vi "TryUpdateGyroSBIT.vi"   [LabVIEW 2018]
uses:
  <vilib>/Platform/TimedLoop/XDataNode/timing_clust.ctl
  <vilib>/Platform/TimedLoop/XDataNode/nitl_modes.ctl
  <vilib>/Platform/TimedLoop/XDataNode/wakeup.ctl
  Telemetry/TelemetryDataTypes.ctl
  Telemetry/TelemetryUpdateModes.ctl
  Telemetry/TelemetryFields.ctl
  <vilib>/rvi/Emulation/niFpgaEmulationIsFPGAContextNoSignature.vi
  <vilib>/rvi/Emulation/niFpgaSctlEmulationGetInTimedLoop.vi
  <vilib>/rvi/errors/niFpgaSetErrorForExecOnDevCompSimple.vi
  <vilib>/rvi/eio/common/nirviEmuReportErrorAndStop.vi
  <vilib>/rvi/DataTransferAndStorage/Container/Common/niFpgaContainerGetUniqueNameForEmu.vi
  <vilib>/rvi/FIFO/Fifo_Resource/nirvififoEmulationSetSize.vi
  <vilib>/rvi/FIFO/Fifo_Resource/nirviFifoEmulationQueueMgr.vi
  <instcachedir>/0/nirviFifoEmulationQueueMgr_E5CAEC123FF24DC58D834DCA3CDAA9B5.lvgen/nirviFifoEmulationQueueMgr_E5CAEC123FF24DC58D834DCA3CDAA9B5_009.vi
  <vilib>/Utility/error.llb/Clear Errors.vi
  <vilib>/rvi/FIFO/Fifo_Resource/nirvififoEmulationCreateLock.vi
  <vilib>/rvi/Emulation/niFpgaProcessEmulError.vi
  <vilib>/rvi/FIFO/Fifo_Resource/nirvififoEmulationObtainLock.vi
  <vilib>/rvi/FIFO/Fifo_Resource/nirvififoEmulationReleaseLock.vi
  <vilib>/rvi/occurrence/nirviWaitOnOccurrenceBase.vi
  <vilib>/rvi/errors/nirviReportUnexpectedCaseInternalError.vi
  <vilib>/rvi/errors/nirviReportUnexpectedCaseInternalError (U32).vi
  <vilib>/rvi/Emulation/niFpgaEmulationReportErrorSimple.vi
  <vilib>/rvi/Emulation/niFpgaGetClockAttributes.vi
  <vilib>/rvi/Emulation/niFpgaCriticalErrorInLSC.vi
  <instcachedir>/0/nirviFifoEmulationQueueMgr_E5CAEC123FF24DC58D834DCA3CDAA9B5.lvgen/nirviFifoEmulationQueueMgr_E5CAEC123FF24DC58D834DCA3CDAA9B5_007.vi
  <vilib>/rvi/FIFO/Fifo_Resource/nirvififoEmulationDetermineInputValidOut.vi
  <vilib>/rvi/Memory/Memory_Emulation/niFpgaMemoryEmulationCacheClearOnFirstRun.vi
  <vilib>/rvi/Memory/Memory_Emulation/nirvimemoryEmulationManagerCache_MakeExclusive.vi
  <vilib>/rvi/Memory/Memory_Emulation/niFpgaMemoryEmulationValidateCache.vi
  <vilib>/rvi/Memory/Memory_Emulation/nirvimemoryEmulationManagerCache_InsertValue.vi
  <vilib>/rvi/Memory/Memory_Emulation/nirvimemoryEmulationManagerCache_ReleaseExclusive.vi
  <vilib>/rvi/Memory/Memory_Emulation/nirvimemoryEmulationManagerCache_GetValue.vi
  <vilib>/rvi/Memory/Memory_Emulation/nirvimemoryEmulationManagerCache_SetValue.vi
  <vilib>/rvi/DataTransferAndStorage/Container/XNode/niFpgaContainer.xnode
  <vilib>/rvi/FIFO/Fifo_Resource/nirvififoEmulationRead.vi
  <vilib>/Platform/TimedLoop/XDataNode/XDataNode.xnode
  <vilib>/rvi/FIFO/Fifo_Resource/nirvififoEmulationWrite.vi
  <vilib>/rvi/DataTransferAndStorage/Register/Emulation/niFpgaRegisterEmulation.vi
  <vilib>/Platform/TimedLoop/XDataNode/XDNodeRunTimeDep.lvlib
types:
  T1 = cluster{"Timestamp":u64, "TxBytes":u64, "RxBytes":u64, "TxFrames":u64, "RxFrames":u64, "BIT0":u8, "BIT1":u8, "BIT2":u8, "BIT3":u8, "BIT4":u8, "BIT5":u8}
  T2 = typedef "TelemetryFields.ctl" = enum16{"None", "InclinometerTxBytes", "InclinometerRxBytes", "InclinometerTxFrames", "InclinometerRxFrames", "InclinometerErrorTimestamp", "InclinometerErrorCode", "InclinometerSampleTimestamp", "InclinometerAngleRaw", "DisplacementTxBytes", "DisplacementRxBytes", "DisplacementTxFrames", "DisplacementRxFrames", "DisplacementErrorTimestamp", "DisplacementErrorCode", "DisplacementSampleTimestamp", "DisplacementRaw1", "DisplacementRaw2", "DisplacementRaw3", "DisplacementRaw4", "DisplacementRaw5", "DisplacementRaw6", "DisplacementRaw7", "DisplacementRaw8", "AccelerometerSampleCount", "AccelerometerSampleTimestamp", "AccelerometerRaw1", "AccelerometerRaw2", "AccelerometerRaw3", "AccelerometerRaw4", "AccelerometerRaw5", "AccelerometerRaw6", "AccelerometerRaw7", "AccelerometerRaw8", "GyroTxBytes", "GyroRxBytes", "GyroTxFrames", "GyroRxFrames", "GyroErrorTimestamp", "GyroErrorCode", "GyroSampleTimestamp", "GyroRawX", "GyroRawY", "GyroRawZ", "GyroStatus", "GyroSequenceNumber", "GyroTemperature", "GyroBITTimestamp", "GyroBIT0", "GyroBIT1", "GyroBIT2", "GyroBIT3", "GyroBIT4", "GyroBIT5", "GyroBIT6", "GyroBIT7", "DigitalInputSampleCount", "DigitalInputTimestamp", "DigitalInputStates", "DigitalOutputSampleCount", "DigitalOutputTimestamp", "DigitalOutputStates", "PowerSupplySampleCount", "PowerSupplyTimestamp", "PowerSupplyStates", "Modbus1ErrorFlags", "Modbus1TxByteCount", "Modbus1TxFrameCount", "Modbus1RxByteCount", "Modbus1RxFrameCount", "Modbus2ErrorFlags", "Modbus2TxByteCount", "Modbus2TxFrameCount", "Modbus2RxByteCount", "Modbus2RxFrameCount", "Modbus3ErrorFlags", "Modbus3TxByteCount", "Modbus3TxFrameCount", "Modbus3RxByteCount", "Modbus3RxFrameCount", "Modbus4ErrorFlags", "Modbus4TxByteCount", "Modbus4TxFrameCount", "Modbus4RxByteCount", "Modbus4RxFrameCount"}
  T3 = typedef "TelemetryUpdateModes.ctl" = enum8{"=", "+", "-", "|"}
  T4 = typedef "TelemetryDataTypes.ctl" = enum8{"U8", "U16", "U32", "U64", "I8", "I16", "I32", "I64", "SGL"}
  T5 = typedef "XDNodeRunTimeDep.lvlib/timing_clust.ctl" = cluster{"Expected End [f-1]":u64, "Actual End [f-1]":u64, "Finished Late? [f-1]":bool, "Expected End [i-1]":u64, "Actual End [i-1]":u64, "Finished Late? [i-1]":bool, "Expected Start [i]":u64, "Actual Start [i]":u64, "Expected Start [f]":u64, "Actual Start [f]":u64, "Source Name":string, "Structure Name":string, "Period":i64, "Deadline":i64, "Offset":i64, "Start":i64, "Priority":i32, "Timeout":i32, "Mode":T6, "Wakeup Reason":T7, "Error":errorcluster, "Source Type":string, "Secondary Source Type":string, "Global End Time":u64, "Global Start Time":u64, "Frame Duration":u64, "Iteration Duration":u64, "Assigned CPU":i32, "I/O Scan Engine Mode":u32}
  T6 = typedef "XDNodeRunTimeDep.lvlib/nitl_modes.ctl" = enum32{"No Change", "Process missed periods, maintain original phase", "Discard missed periods, maintain original phase", "Process missed periods, ignore original phase", "Discard missed periods, ignore original phase"}
  T7 = typedef "XDNodeRunTimeDep.lvlib/wakeup.ctl" = enum32{"Normal", "Aborted", "Asynchronous wakeup", "Timing source error", "Timed loop error", "Timeout"}
  T8 = typedef "TelemetryUpdateData.ctl" = cluster{"DataType":T4, "Mode":T3, "Field":T2, "Data":u64}
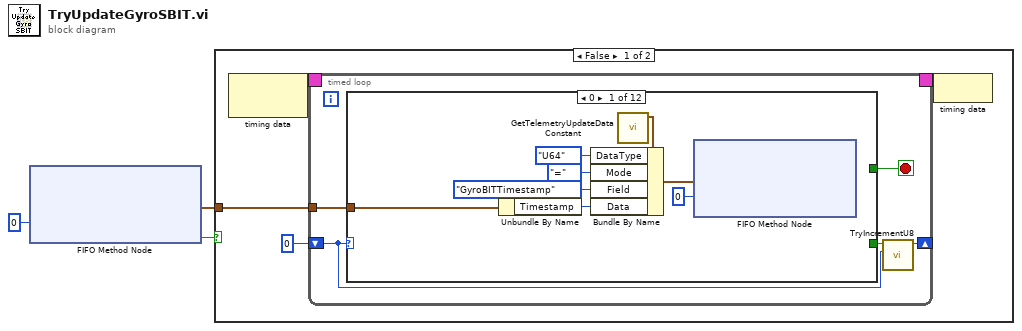
[diagram p0: block diagram]
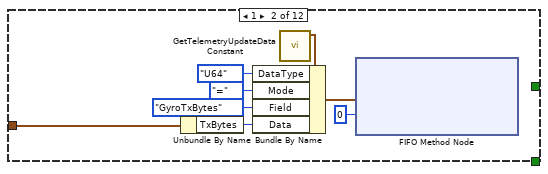
[diagram p2: hidden frame]
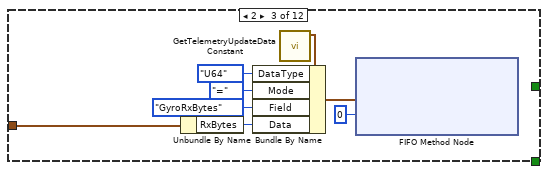
[diagram p3: hidden frame]
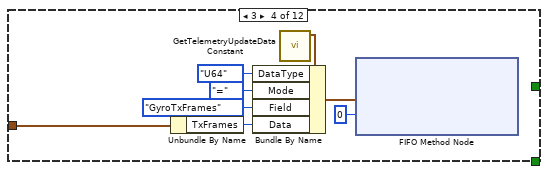
[diagram p4: hidden frame]
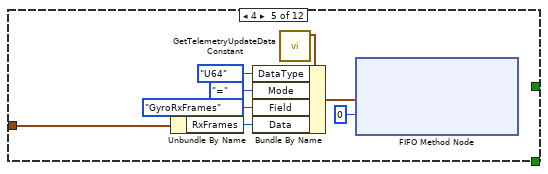
[diagram p5: hidden frame]
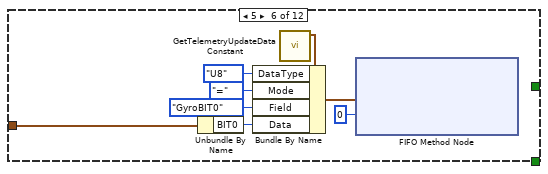
[diagram p6: hidden frame]
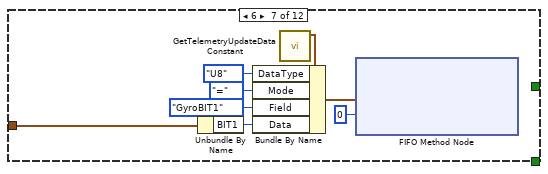
[diagram p7: hidden frame]
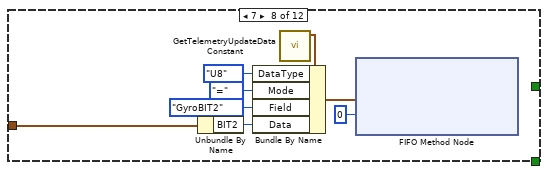
[diagram p8: hidden frame]
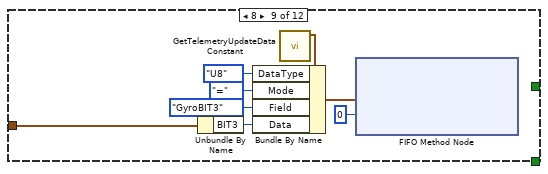
[diagram p9: hidden frame]
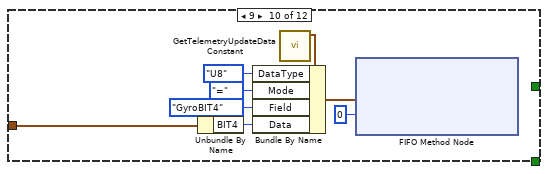
[diagram p10: hidden frame]
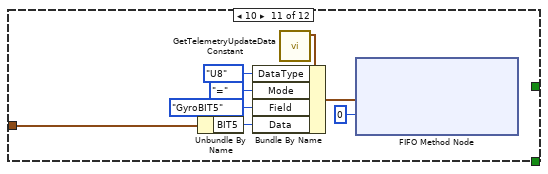
[diagram p11: hidden frame]
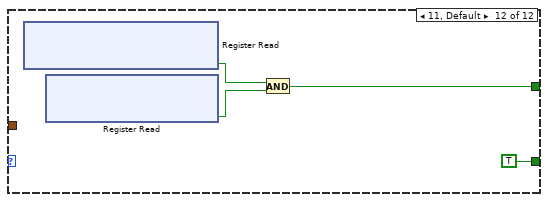
[diagram p12: hidden frame]
diagram:
  n1 = xnode ("FIFO Method Node")("Timeout"=0) -> ("Element"=w1:T1, "Timed Out?"=w2:bool)  [unwired: 1 in, 1 out]
  n2 = case shown="False" w2 {
    tunnel: w1 -> [w7 _]
    frame False {
      n3 = node-c288() -> (w6:T5)  [unwired: 1 in]
      n4 = timed-loop {
        tunnel: w7 -> [w12]
        timing: w6 -> [_]
        timing-out: [_] -> w5
        shift-right: [w10] -> _
        shift-left: u8 0 -> [w9]
        stop <- w11 stop-if-true
        n5 = case shown="0" w9 {
          tunnel: w12 -> [w13 w21 w29 w37 w45 w53 w61 w69 w77 w85 w93 _]
          tunnel: [_ _ _ _ _ _ _ _ _ _ _ w102] -> w11
          tunnel: [_ _ _ _ _ _ _ _ _ _ _ TRUE] -> w8
          frame 0 {
            n6 = Unbundle By Name(w13) -> ("Timestamp"=w19:u64)
            n7 = call "GetTelemetryUpdateDataConstant.vi"() -> ("TelemetryUpdateData"=w18:T8)  [unwired: 11 in]
            n8 = Bundle By Name(cluster=w18, "DataType"=TelemetryDataTypes."U64", "Mode"=TelemetryUpdateModes."=", "Field"=TelemetryFields."GyroBITTimestamp" ("TelemetryFields"), "Data"=w19) -> (w15:T8)
            n9 = xnode ("FIFO Method Node")("Element"=w15, "Timeout"=0) -> ()  [unwired: 1 in, 2 out]
          }
          frame 1 {
            n10 = Unbundle By Name(w21) -> ("TxBytes"=w22:u64)
            n11 = call "GetTelemetryUpdateDataConstant.vi"() -> ("TelemetryUpdateData"=w23:T8)  [unwired: 11 in]
            n12 = Bundle By Name(cluster=w23, "DataType"=TelemetryDataTypes."U64", "Mode"=TelemetryUpdateModes."=", "Field"=TelemetryFields."GyroTxBytes", "Data"=w22) -> (w27:T8)
            n13 = xnode ("FIFO Method Node")("Element"=w27, "Timeout"=0) -> ()  [unwired: 1 in, 2 out]
          }
          frame 2 {
            n14 = Unbundle By Name(w29) -> ("RxBytes"=w36:u64)
            n15 = call "GetTelemetryUpdateDataConstant.vi"() -> ("TelemetryUpdateData"=w35:T8)  [unwired: 11 in]
            n16 = Bundle By Name(cluster=w35, "DataType"=TelemetryDataTypes."U64", "Mode"=TelemetryUpdateModes."=", "Field"=TelemetryFields."GyroRxBytes", "Data"=w36) -> (w31:T8)
            n17 = xnode ("FIFO Method Node")("Element"=w31, "Timeout"=0) -> ()  [unwired: 1 in, 2 out]
          }
          frame 3 {
            n18 = Unbundle By Name(w37) -> ("TxFrames"=w38:u64)
            n19 = call "GetTelemetryUpdateDataConstant.vi"() -> ("TelemetryUpdateData"=w39:T8)  [unwired: 11 in]
            n20 = Bundle By Name(cluster=w39, "DataType"=TelemetryDataTypes."U64", "Mode"=TelemetryUpdateModes."=", "Field"=TelemetryFields."GyroTxFrames", "Data"=w38) -> (w43:T8)
            n21 = xnode ("FIFO Method Node")("Element"=w43, "Timeout"=0) -> ()  [unwired: 1 in, 2 out]
          }
          frame 4 {
            n22 = Unbundle By Name(w45) -> ("RxFrames"=w52:u64)
            n23 = call "GetTelemetryUpdateDataConstant.vi"() -> ("TelemetryUpdateData"=w51:T8)  [unwired: 11 in]
            n24 = Bundle By Name(cluster=w51, "DataType"=TelemetryDataTypes."U64", "Mode"=TelemetryUpdateModes."=", "Field"=TelemetryFields."GyroRxFrames", "Data"=w52) -> (w47:T8)
            n25 = xnode ("FIFO Method Node")("Element"=w47, "Timeout"=0) -> ()  [unwired: 1 in, 2 out]
          }
          frame 5 {
            n26 = Unbundle By Name(w53) -> ("BIT0"=w54:u8)
            n27 = call "GetTelemetryUpdateDataConstant.vi"() -> ("TelemetryUpdateData"=w55:T8)  [unwired: 11 in]
            n28 = Bundle By Name(cluster=w55, "DataType"=TelemetryDataTypes."U8", "Mode"=TelemetryUpdateModes."=", "Field"=TelemetryFields."GyroBIT0" ("TelemetryFields"), "Data"=w54) -> (w58:T8)
            n29 = xnode ("FIFO Method Node")("Element"=w58, "Timeout"=0) -> ()  [unwired: 1 in, 2 out]
          }
          frame 6 {
            n30 = Unbundle By Name(w61) -> ("BIT1"=w62:u8)
            n31 = call "GetTelemetryUpdateDataConstant.vi"() -> ("TelemetryUpdateData"=w63:T8)  [unwired: 11 in]
            n32 = Bundle By Name(cluster=w63, "DataType"=TelemetryDataTypes."U8", "Mode"=TelemetryUpdateModes."=", "Field"=TelemetryFields."GyroBIT1" ("TelemetryFields"), "Data"=w62) -> (w66:T8)
            n33 = xnode ("FIFO Method Node")("Element"=w66, "Timeout"=0) -> ()  [unwired: 1 in, 2 out]
          }
          frame 7 {
            n34 = Unbundle By Name(w69) -> ("BIT2"=w70:u8)
            n35 = call "GetTelemetryUpdateDataConstant.vi"() -> ("TelemetryUpdateData"=w71:T8)  [unwired: 11 in]
            n36 = Bundle By Name(cluster=w71, "DataType"=TelemetryDataTypes."U8", "Mode"=TelemetryUpdateModes."=", "Field"=TelemetryFields."GyroBIT2" ("TelemetryFields"), "Data"=w70) -> (w74:T8)
            n37 = xnode ("FIFO Method Node")("Element"=w74, "Timeout"=0) -> ()  [unwired: 1 in, 2 out]
          }
          frame 8 {
            n38 = Unbundle By Name(w77) -> ("BIT3"=w78:u8)
            n39 = call "GetTelemetryUpdateDataConstant.vi"() -> ("TelemetryUpdateData"=w79:T8)  [unwired: 11 in]
            n40 = Bundle By Name(cluster=w79, "DataType"=TelemetryDataTypes."U8", "Mode"=TelemetryUpdateModes."=", "Field"=TelemetryFields."GyroBIT3" ("TelemetryFields"), "Data"=w78) -> (w82:T8)
            n41 = xnode ("FIFO Method Node")("Element"=w82, "Timeout"=0) -> ()  [unwired: 1 in, 2 out]
          }
          frame 9 {
            n42 = Unbundle By Name(w85) -> ("BIT4"=w86:u8)
            n43 = call "GetTelemetryUpdateDataConstant.vi"() -> ("TelemetryUpdateData"=w87:T8)  [unwired: 11 in]
            n44 = Bundle By Name(cluster=w87, "DataType"=TelemetryDataTypes."U8", "Mode"=TelemetryUpdateModes."=", "Field"=TelemetryFields."GyroBIT4" ("TelemetryFields"), "Data"=w86) -> (w90:T8)
            n45 = xnode ("FIFO Method Node")("Element"=w90, "Timeout"=0) -> ()  [unwired: 1 in, 2 out]
          }
          frame 10 {
            n46 = Unbundle By Name(w93) -> ("BIT5"=w94:u8)
            n47 = call "GetTelemetryUpdateDataConstant.vi"() -> ("TelemetryUpdateData"=w95:T8)  [unwired: 11 in]
            n48 = Bundle By Name(cluster=w95, "DataType"=TelemetryDataTypes."U8", "Mode"=TelemetryUpdateModes."=", "Field"=TelemetryFields."GyroBIT5" ("TelemetryFields"), "Data"=w94) -> (w98:T8)
            n49 = xnode ("FIFO Method Node")("Element"=w98, "Timeout"=0) -> ()  [unwired: 1 in, 2 out]
          }
          frame 11, Default {
            n50 = xnode ("Register Read")() -> ("Data"=w104:bool)  [unwired: 1 in, 1 out]
            n51 = xnode "Register Read"() -> ("Data"=w103:bool)  [unwired: 1 in, 1 out]
            n52 = And(x=w104, y=w103) -> (x .and. y?=w102:bool)
          }
        }
        n53 = call "TryIncrementU8.vi"("In"=w9, "DontInc"=w8) -> ("Out"=w10:u8)  [unwired: 9 in]
      }
      n54 = node-c288(w5) -> ()
    }
    frame True {
    }
  }
